vi "ROI entry-Trig delay sanity check.vi"(8 "error in (no error)":errorcluster) -> (0 "error out":errorcluster, 3 "Trigger delay is valid":bool)   [LabVIEW 2017]
uses:
  ROI Entry screen/Globals/gl_ROI Entry UI globals.vi
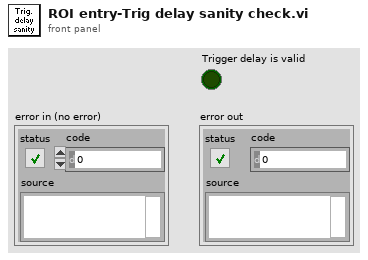
[diagram p1: front panel]
types:
  T1 = typedef "ROI entry screen ctrl refs cluster.ctl" = cluster{"Done button":refnum<vi>, "Imaging button":refnum<vi>, "Acquisition button":refnum<vi>, "POI dwell time (us)":refnum<vi>, "Scan dwell time per pixel (us)":refnum<vi>, "# of planes":refnum<vi>, "Zoom Ctrl":refnum<vi>, "Equal size":refnum<vi>, "Channel":refnum<vi>, "Image Display":refnum<vi>, "Z-Plane Selector":refnum<vi>, "Number of lines left":refnum<vi>, "Z-stack folder path":refnum<vi>, "POI Density":refnum<vi>, "Arb Plane Entry":refnum<vi>, "Whole plane":refnum<vi>, "Clear Last":refnum<vi>, "Clear All":refnum<vi>, "Trial Length (sec)":refnum<vi>, "Palette Type":refnum<vi>, "Intensity slider":refnum<vi>, "# POI":refnum<vi>, "Max Z Proj":refnum<vi>, "Zplane ind":refnum<vi>, "Wavelength (nm)":refnum<vi>, "Number of Trials":refnum<vi>, "Funct stim.trig.enable":refnum<vi>, "Funct stim.trig.delay (s)":refnum<vi>, "Line Mode":refnum<vi>, "Step size (µm)":refnum<vi>, "ROI move mode":refnum<vi>, "Cool-down time (s)":refnum<vi>, "Enable cool-down time":refnum<vi>, "Motor Z ind. (um)":refnum<vi>, "AOL Z ind. (um)":refnum<vi>, "Load Reference Image":refnum<vi>}
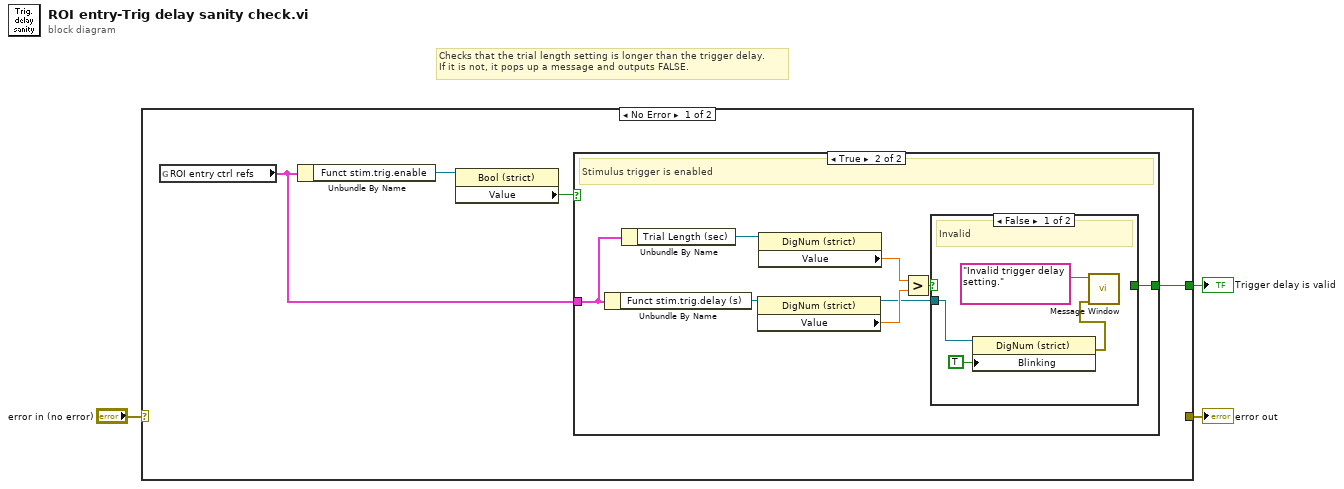
[diagram p0: block diagram]
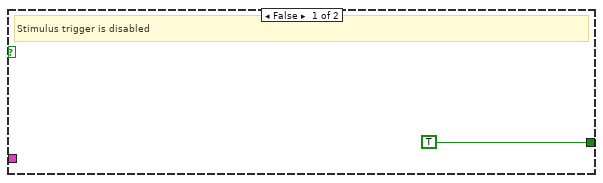
[diagram p2: hidden frame]
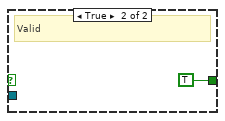
[diagram p3: hidden frame]
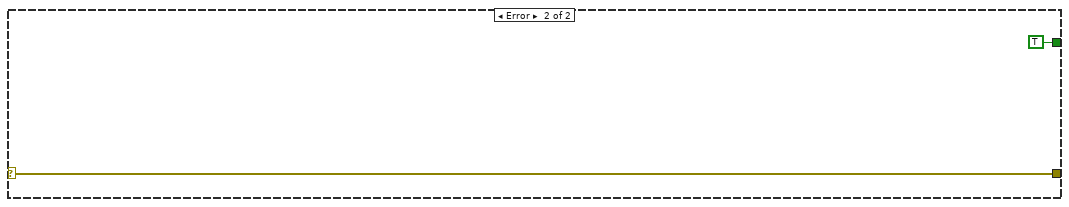
[diagram p4: hidden frame]
diagram:
  # "Checks that the trial length setting is longer than the trigger delay.\nIf it is not, it pops up a message and outputs FALSE."
  n1 = case shown="No Error" "error in (no error)" {
    selector: "error in (no error)" -> [_ w23]
    tunnel: [w4 TRUE] -> w3
    tunnel: [_ w23] -> w1
    frame No Error {
      n2 = global read "gl_ROI Entry UI globals.vi" "ROI entry ctrl refs"() -> (w7:T1)
      n3 = Unbundle By Name(w7) -> ("Funct stim.trig.enable"=w6:refnum<vi>)
      n4 = property on="Property Node" class="Bool (strict)"(reference=w6) -> ("Value"=w5:bool)  [unwired: 1 in, 2 out]
      n5 = case shown="True" w5 {
        tunnel: w7 -> [_ w14]
        tunnel: [TRUE w10] -> w4
        frame False {
          # "Stimulus trigger is disabled"
        }
        frame True {
          # "Stimulus trigger is enabled"
          n6 = Unbundle By Name(w14) -> ("Funct stim.trig.delay (s)"=w16:refnum<vi>)
          n7 = Unbundle By Name(w14) -> ("Trial Length (sec)"=w15:refnum<vi>)
          n8 = property on="Property Node" class="DigNum (strict)"(reference=w16) -> (reference out=w9:refnum<vi>, "Value"=w12:dbl)  [unwired: 1 in, 1 out]
          n9 = property on="Property Node" class="DigNum (strict)"(reference=w15) -> ("Value"=w13:dbl)  [unwired: 1 in, 2 out]
          n10 = Greater?(x=w13, y=w12) -> (0:w11:bool)
          n11 = case shown="False" w11 {
            tunnel: [_ TRUE] -> w10
            tunnel: w9 -> [w19 _]
            frame False {
              # "Invalid"
              n12 = property on="Property Node" class="DigNum (strict)"(reference=w19, "Blinking"=TRUE) -> (error out=w17:errorcluster)  [unwired: 1 in, 1 out]
              n13 = call "Message Window.vi"("error in (no error)"=w17, "Message string"="Invalid trigger delay setting.") -> ()  [unwired: 9 in, 1 out]
            }
            frame True {
              # "Valid"
            }
          }
        }
      }
    }
    frame Error {
    }
  }
  "error out" <- w1
  "Trigger delay is valid" <- w3
